vi "RangeI2C-loop.vi"(0 "Remote IP Address":string="192.168.124.53", 1 "Remote Port":u16=502, 2 "I2C Operation Control":T1(ring)=enum."Command Find Range", 3 "SCL DIO Ch. No.":u16=2, 4 "SDA DIO Ch. No.":u16=3, 5 "CURRENT 8-bit address (dec.)":u16=224, 8 "NEW 8-bit address (dec.)":u8=224) -> (6 "Range (cm)":dbl=27.0, 7 "Range (in.)":dbl=10.62992125984252)   [LabVIEW 2014]
panel:
  out "Waveform Graph":dbl[](graph)=[38.0, 38.0, 38.0, 38.0, 27.0, 27.0, 27.0, 27.0, 27.0, 27.0, 27.0, 27.0, 27.0, 27.0, 27.0, 27.0, 27.0, 27.0, 27.0, 27.0, 27.0, 27.0, 27.0, 27.0, 27.0, 27.0, 27.0, 27.0, 27.0, 27.0, 27.0, 27.0, 27.0, 27.0, 27.0, 27.0, 27.0]
  in  "stop":bool
  # "Even address values up to 254\n\nInvalid Address Values: 0, 80, 164, 170"
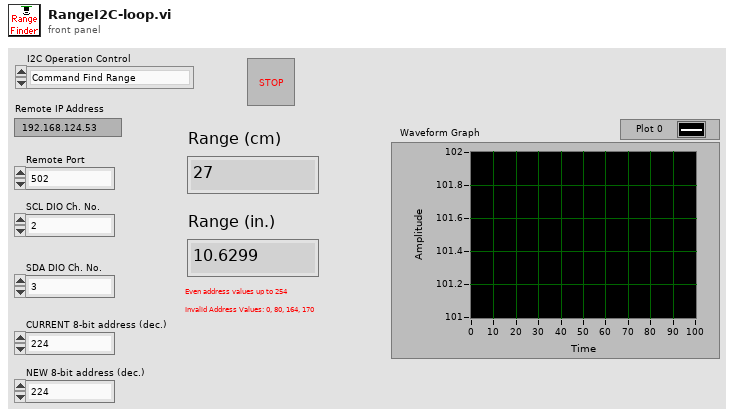
[diagram p1: front panel]
types:
  T1 = enum16{"Configure I2C Settings", "Command Find Range", "Command Read Range", "Report the last range value", "Change sensor address", "Wait to range 100ms"}
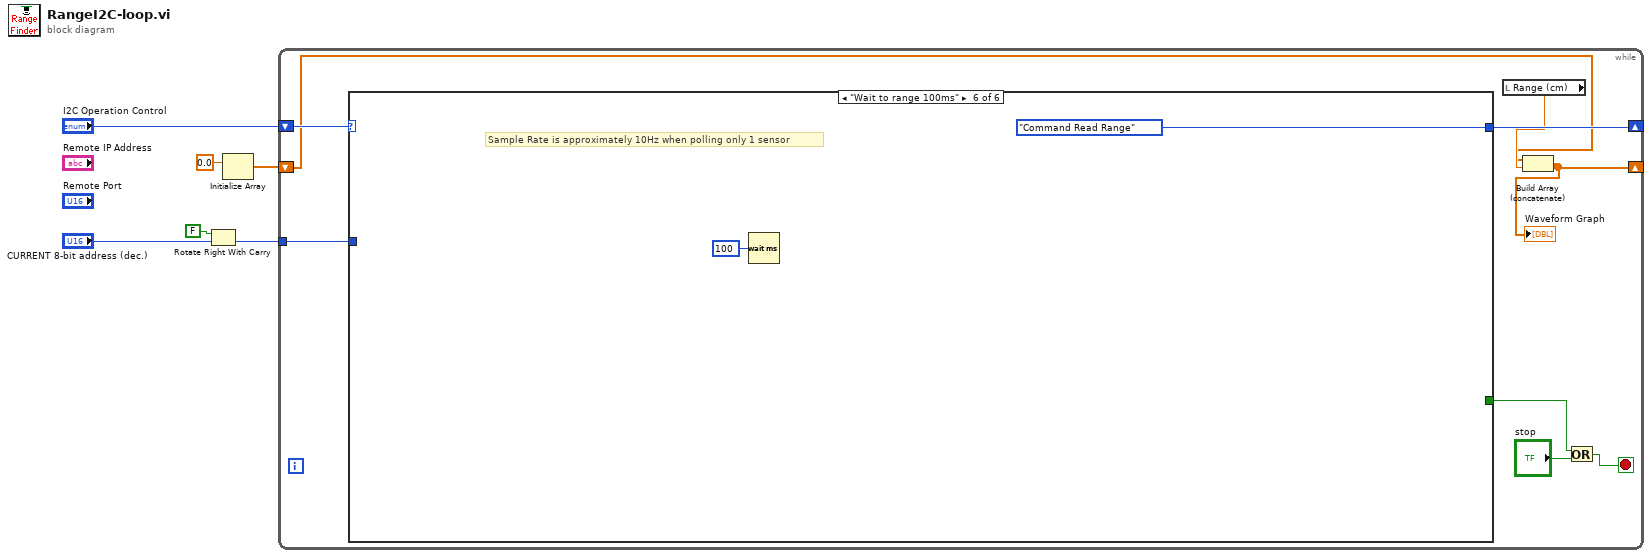
[diagram p0: block diagram]
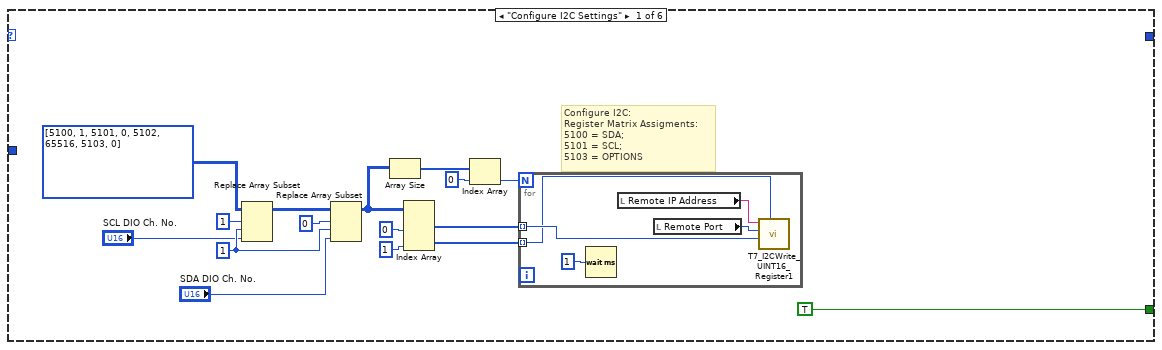
[diagram p2: hidden frame]
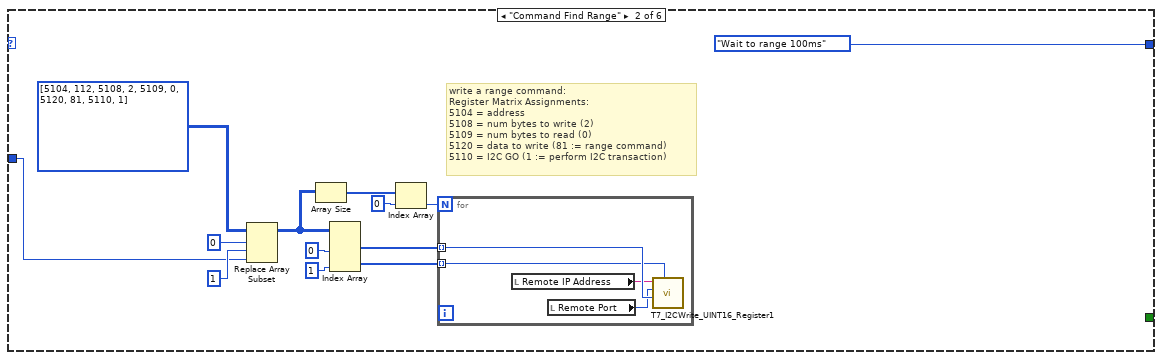
[diagram p3: hidden frame]
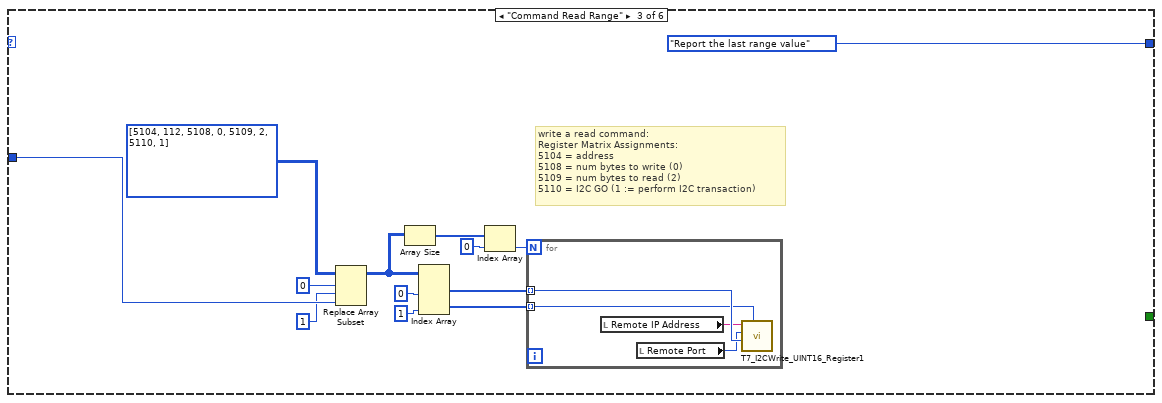
[diagram p4: hidden frame]
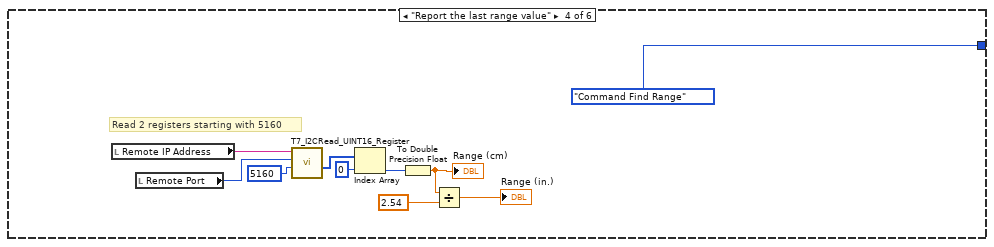
[diagram p5: hidden frame]
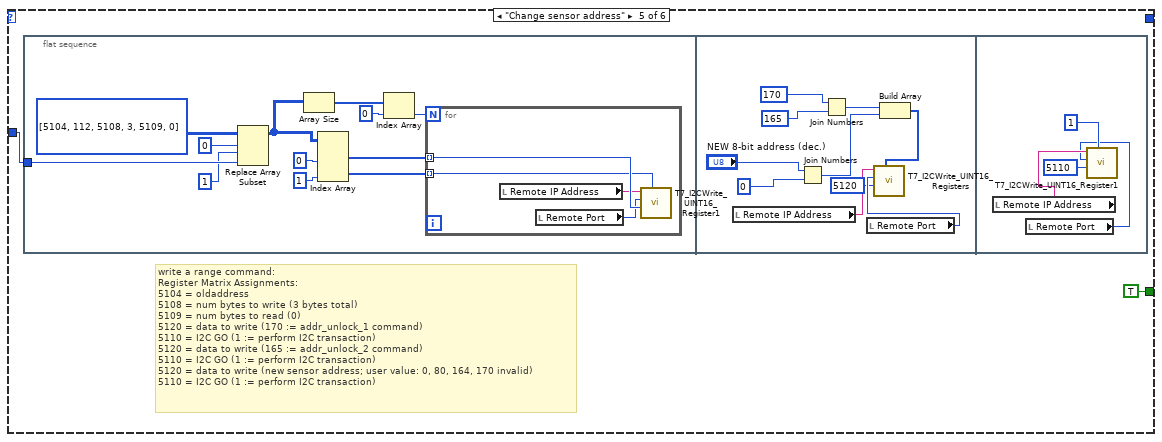
[diagram p6: hidden frame]
diagram:
  n1 = Rotate Right With Carry(2:"CURRENT 8-bit address (dec.)", 3:FALSE ("carry")) -> (0:w3:u16)  [unwired: 1 out]
  n2 = Initialize Array(0.0 ("element")) -> (w2:dbl[])  [unwired: 1 in]
  n3 = while {
    tunnel: w3 -> [w15]
    shift-right: [w14] -> _
    shift-left: "I2C Operation Control" -> [w10]
    shift-right: [w8] -> _
    shift-left: w2 -> [w7]
    stop <- w11 stop-if-true
    n4 = case shown="\"Wait to range 100ms\"" w10 {
      tunnel: w15 -> [_ w39 w66 _ w82 _]
      tunnel: [_ T1."Wait to range 100ms" ("I2C Operation Control") T1."Report the last range value" ("I2C Operation Control") T1."Command Find Range" ("I2C Operation Control") _ T1."Command Read Range" ("I2C Operation Control")] -> w14
      tunnel: [TRUE ("x") _ _ _ TRUE ("x") _] -> w12
      frame "Configure I2C Settings" {
        w21 = 1 ("disabled index (col)")
        # "Configure I2C: \nRegister Matrix Assigments:\n5100 = SDA;\n5101 = SCL;\n5103 = OPTIONS"
        n5 = Replace Array Subset(array=i32[][] [[5100, 1], [5101, 0], [5102, 65516], [5103, 0]], new element="SCL DIO Ch. No.", index (row)=1, index (col)=w21) -> (w20:i32[][])
        n6 = Replace Array Subset(array=w20, new element="SDA DIO Ch. No.", index (row)=0, index (col)=w21) -> (w17:i32[][])
        n7 = Array Size(array=w17) -> (size(s)=w31:i32[])
        n8 = Index Array(array=w17, index (col) #1=0 ("disabled index (col)"), index (col) #2=1 ("index (col)")) -> (element #1=w26:i32[], element #2=w25:i32[])  [unwired: 2 in]
        n9 = Index Array(array=w31, index=0) -> (element=w29:i32)
        n10 = for {
          N: w29 -> [_]
          tunnel: w26 -> [w36] mode=indexing
          tunnel: w25 -> [w35] mode=indexing
          n11 = Wait (ms)(milliseconds to wait=u32 1) -> ()  [unwired: 1 out]
          n12 = local read "Remote IP Address"() -> (w34:string)
          n13 = local read "Remote Port"() -> (w33:u16)
          n14 = call "T7_I2CWrite_UINT16_Register1.vi"("Remote IP Address"=w34, "Remote Port"=w33, "Starting Address"=w36, "UINT16 to Write"=w35) -> ()  [unwired: 5 in, 2 out]
        }
      }
      frame "Command Find Range" {
        # "write a range command:\nRegister Matrix Assignments:\n5104 = address\n5108 = num bytes to write (2)\n5109 = num bytes to read (0)\n5120 = data to write (81 := range command)\n5110 = I2C GO (1 := perform I2C transaction)"
        n15 = Replace Array Subset(array=i32[][] [[5104, 112], [5108, 2], [5109, 0], [5120, 81], [5110, 1]], new element=w39, index (row)=0, index (col)=1 ("disabled index (col)")) -> (w38:i32[][])
        n16 = Array Size(array=w38) -> (size(s)=w49:i32[])
        n17 = Index Array(array=w38, index (col) #1=0 ("disabled index (col)"), index (col) #2=1 ("index (col)")) -> (element #1=w44:i32[], element #2=w43:i32[])  [unwired: 2 in]
        n18 = Index Array(array=w49, index=0) -> (element=w47:i32)
        n19 = for {
          N: w47 -> [_]
          tunnel: w44 -> [w53] mode=indexing
          tunnel: w43 -> [w52] mode=indexing
          n20 = local read "Remote IP Address"() -> (w51:string)
          n21 = local read "Remote Port"() -> (w50:u16)
          n22 = call "T7_I2CWrite_UINT16_Register1.vi"("Remote IP Address"=w51, "Remote Port"=w50, "Starting Address"=w53, "UINT16 to Write"=w52) -> ()  [unwired: 5 in, 2 out]
        }
      }
      frame "Command Read Range" {
        # "write a read command:\nRegister Matrix Assignments:\n5104 = address\n5108 = num bytes to write (0)\n5109 = num bytes to read (2)\n5110 = I2C GO (1 := perform I2C transaction)"
        n23 = Replace Array Subset(array=i32[][] [[5104, 112], [5108, 0], [5109, 2], [5110, 1]], new element=w66, index (row)=0, index (col)=1 ("disabled index (col)")) -> (w54:i32[][])
        n24 = Array Size(array=w54) -> (size(s)=w55:i32[])
        n25 = Index Array(array=w54, index (col) #1=0 ("disabled index (col)"), index (col) #2=1 ("index (col)")) -> (element #1=w60:i32[], element #2=w61:i32[])  [unwired: 2 in]
        n26 = Index Array(array=w55, index=0) -> (element=w57:i32)
        n27 = for {
          N: w57 -> [_]
          tunnel: w60 -> [w70] mode=indexing
          tunnel: w61 -> [w69] mode=indexing
          n28 = local read "Remote IP Address"() -> (w68:string)
          n29 = local read "Remote Port"() -> (w67:u16)
          n30 = call "T7_I2CWrite_UINT16_Register1.vi"("Remote IP Address"=w68, "Remote Port"=w67, "Starting Address"=w70, "UINT16 to Write"=w69) -> ()  [unwired: 5 in, 2 out]
        }
      }
      frame "Report the last range value" {
        # "Read 2 registers starting with 5160"
        n31 = local read "Remote IP Address"() -> (w78:string)
        n32 = local read "Remote Port"() -> (w79:u16)
        n33 = call "T7_I2CRead_UINT16_Register.vi"("FirstChannel"=5160, "Remote Port"=w79, "Remote IP Address"=w78) -> ("Raw Data Read"=w77:u16[])  [unwired: 6 in, 2 out]
        n34 = Index Array(array=w77, index=0) -> (element=w75:u16)
        n35 = To Double Precision Float(number=w75) -> (double precision float=w71:dbl)
        "Range (cm)" <- w71
        n36 = Divide(x=w71, y=2.54) -> (x/y=→"Range (in.)":dbl)
      }
      frame "Change sensor address" {
        # "write a range command:\nRegister Matrix Assignments:\n5104 = oldaddress\n5108 = num bytes to write (3 bytes total)\n5109 = num bytes to read (0)\n5120 = data to write (170 := addr_unlock_1 command)\n5110 = I2C GO (1 := perform I2C transaction)\n5120 = data to write (165 := addr_unlock_2 command)\n5110 = I2C GO (1 := perform I2C transaction)\n5120 = data to write (new sensor address; user value: 0, 80, 164, 170 invalid)\n5110 = I2C GO (1 := perform I2C transaction)"
        n37 = flat-sequence {
          tunnel: w82 -> [w85]
          frame #0 {
            n38 = Replace Array Subset(array=i32[][] [[5104, 112], [5108, 3], [5109, 0]], new element=w85, index (row)=0, index (col)=1 ("disabled index (col)")) -> (w83:i32[][])
            n39 = Array Size(array=w83) -> (size(s)=w94:i32[])
            n40 = Index Array(array=w83, index (col) #1=0 ("disabled index (col)"), index (col) #2=1 ("index (col)")) -> (element #1=w89:i32[], element #2=w88:i32[])  [unwired: 2 in]
            n41 = Index Array(array=w94, index=0) -> (element=w92:i32)
            n42 = for {
              N: w92 -> [_]
              tunnel: w89 -> [w98] mode=indexing
              tunnel: w88 -> [w97] mode=indexing
              n43 = local read "Remote IP Address"() -> (w96:string)
              n44 = local read "Remote Port"() -> (w95:u16)
              n45 = call "T7_I2CWrite_UINT16_Register1.vi"("Remote IP Address"=w96, "Remote Port"=w95, "Starting Address"=w98, "UINT16 to Write"=w97) -> ()  [unwired: 5 in, 2 out]
            }
          }
          frame #1 {
            n46 = local read "Remote IP Address"() -> (w101:string)
            n47 = Join Numbers(hi="NEW 8-bit address (dec.)", lo=u8 0) -> ((hi.lo)=w103:u16)
            n48 = Join Numbers(hi=u8 170, lo=u8 165) -> ((hi.lo)=w104:u16)
            n49 = local read "Remote Port"() -> (w100:u16)
            n50 = Build Array(w104, w103) -> (w102:u16[])
            n51 = call "T7_I2CWrite_UINT16_Registers.vi"("Remote IP Address"=w101, "Remote Port"=w100, "Starting Address"=u16 5120, "UINT16 to Write"=w102) -> ()  [unwired: 5 in, 2 out]
          }
          frame #2 {
            n52 = local read "Remote IP Address"() -> (w110:string)
            n53 = local read "Remote Port"() -> (w109:u16)
            n54 = call "T7_I2CWrite_UINT16_Register1.vi"("Remote IP Address"=w110, "Remote Port"=w109, "Starting Address"=u16 5110, "UINT16 to Write"=u16 1) -> ()  [unwired: 5 in, 2 out]
          }
        }
      }
      frame "Wait to range 100ms" {
        # "Sample Rate is approximately 10Hz when polling only 1 sensor"
        n55 = Wait (ms)(milliseconds to wait=u32 100) -> ()  [unwired: 1 out]
      }
    }
    n56 = local read "Range (cm)"() -> (w9:dbl)
    n57 = Build Array (concatenate)(w7, w9) -> (w8:dbl[])
    "Waveform Graph" <- w8
    n58 = Or(x=w12, y="stop") -> (x .or. y?=w11:bool)
  }
